vi "Get Boolean.vi"(1 "Name":string) -> (0 "Value":bool)   [LabVIEW 2017, in "Apple script.lvlib"]
doc: "Used to retrieve boolean values for use in \"until\" subcommands."
uses:
  Apple script.lvlib
panel:
  in  "Test Boolean":bool
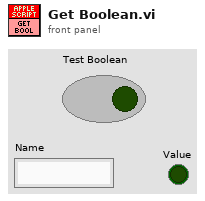
[diagram p1: front panel]
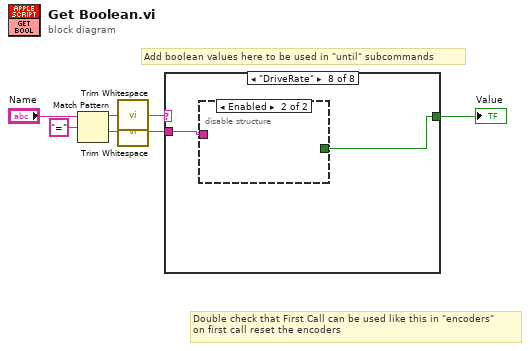
[diagram p0: block diagram]
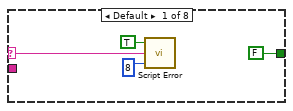
[diagram p2: hidden frame]
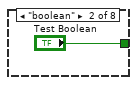
[diagram p3: hidden frame]
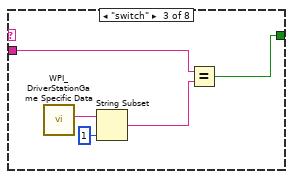
[diagram p4: hidden frame]
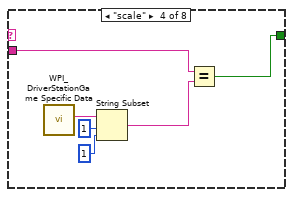
[diagram p5: hidden frame]
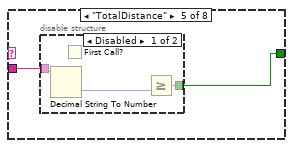
[diagram p6: hidden frame]
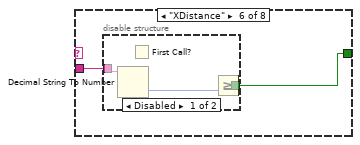
[diagram p8: hidden frame]
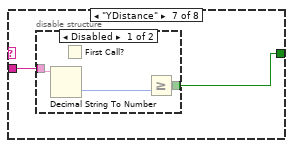
[diagram p10: hidden frame]
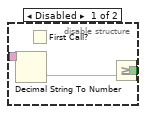
[diagram p12: hidden frame]
diagram:
  # "Double check that First Call can be used like this in \"encoders\"\non first call reset the encoders"
  # "Add boolean values here to be used in \"until\" subcommands"
  n1 = Match Pattern(string="Name", regular expression="=") -> (before substring=w5:string, after substring=w3:string)  [unwired: 1 in, 2 out]
  n2 = call <vilib>:"Trim Whitespace.vi"("string"=w5) -> ("trimmed string"=w2:string)  [unwired: 1 in]
  n3 = call <vilib>:"Trim Whitespace.vi"("string"=w3) -> ("trimmed string"=w1:string)  [unwired: 1 in]
  n4 = case shown="\"DriveRate\"" w2 {
    selector: w2 -> [w8 _ _ _ _ _ _ _]
    tunnel: [FALSE "Test Boolean" w13 w19 w24 w30 w35 w40] -> w7
    tunnel: w1 -> [_ _ w14 w20 w25 w31 w36 w41]
    frame Default {
      n5 = call "Script Error.vi"("Error?"=TRUE, "Error Details"=w8, "Error Code"=8) -> ()  [unwired: 2 in, 1 out]
    }
    frame "boolean" {
    }
    frame "switch" {
      n6 = call <vilib>:"WPI_DriverStationGame Specific Data.vi"() -> ("Game Specific Data"=w17:string)  [unwired: 11 in]
      n7 = String Subset(string=w17, length (rest)=1 ("length (rest)")) -> (substring=w15:string)  [unwired: 1 in]
      n8 = Equal?(x=w14, y=w15) -> (x = y?=w13:bool)
    }
    frame "scale" {
      n9 = call <vilib>:"WPI_DriverStationGame Specific Data.vi"() -> ("Game Specific Data"=w23:string)  [unwired: 11 in]
      n10 = String Subset(string=w23, offset (0)=1, length (rest)=1 ("length (rest)")) -> (substring=w21:string)
      n11 = Equal?(x=w20, y=w21) -> (x = y?=w19:bool)
    }
    frame "TotalDistance" {
      n12 = disable-structure shown="Disabled" {
        disable-tunnel: w25 -> [w28 _]
        disable-tunnel: [w27 _] -> w24
        frame Disabled {
          n13 = Decimal String To Number(string=w28) -> (number=w26:i32)  [unwired: 2 in, 1 out]
          n14 = First Call?() -> ()  [unwired: 1 out]
          n15 = Greater Or Equal?(y=w26) -> (x=w29:i32, x >= y?=w27:bool)
        }
        frame Enabled {
        }
      }
    }
    frame "XDistance" {
      n16 = disable-structure shown="Disabled" {
        disable-tunnel: w31 -> [w34 _]
        disable-tunnel: [w33 _] -> w30
        frame Disabled {
          n17 = Decimal String To Number(string=w34) -> (number=w32:i32)  [unwired: 2 in, 1 out]
          n18 = First Call?() -> ()  [unwired: 1 out]
          n19 = Greater Or Equal?(y=w32) -> (x >= y?=w33:bool)  [unwired: 1 in]
        }
        frame Enabled {
        }
      }
    }
    frame "YDistance" {
      n20 = disable-structure shown="Disabled" {
        disable-tunnel: w36 -> [w39 _]
        disable-tunnel: [w38 _] -> w35
        frame Disabled {
          n21 = Decimal String To Number(string=w39) -> (number=w37:i32)  [unwired: 2 in, 1 out]
          n22 = First Call?() -> ()  [unwired: 1 out]
          n23 = Greater Or Equal?(y=w37) -> (x >= y?=w38:bool)  [unwired: 1 in]
        }
        frame Enabled {
        }
      }
    }
    frame "DriveRate" {
      n24 = disable-structure shown="Enabled" {
        disable-tunnel: w41 -> [w44 _]
        disable-tunnel: [w43 _] -> w40
        frame Disabled {
          n25 = Decimal String To Number(string=w44) -> (number=w42:i32)  [unwired: 2 in, 1 out]
          n26 = First Call?() -> ()  [unwired: 1 out]
          n27 = Greater Or Equal?(y=w42) -> (x >= y?=w43:bool)  [unwired: 1 in]
        }
        frame Enabled {
        }
      }
    }
  }
  "Value" <- w7
